vi "get setpoint.vi"(7 "error in (no error)":errorcluster, 9 "Loop":u8(ring) items=["1", "2", "3", "4"], 10 "VISA In":refnum<visa-resource-name>) -> (0 "error out":errorcluster, 1 "数字":dbl, 3 "VISA out":refnum<visa-resource-name>)   [LabVIEW 2019, in "9T cmag.lvlib"]
uses:
  9T cmag.lvlib
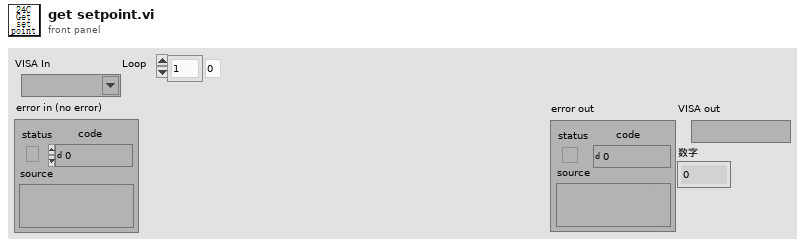
[diagram p1: front panel]
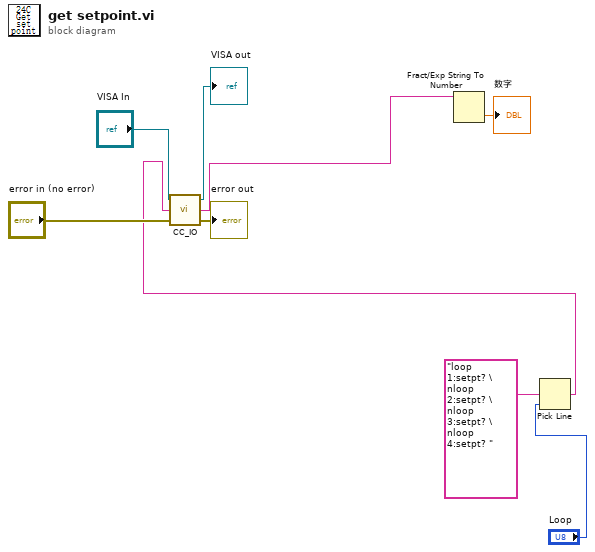
[diagram p0: block diagram]
diagram:
  n1 = Pick Line(multi-line string="loop 1:setpt? \nloop 2:setpt? \nloop 3:setpt? \nloop 4:setpt? " ("string"), line index="Loop") -> (output string=w1:string)  [unwired: 1 in]
  n2 = call "CC_IO.vi"("error in (no error)"="error in (no error)", "Output Command"=w1, "VISA In"="VISA In") -> ("error out"=→"error out":errorcluster, "Input String"=w5:string, "VISA out"=→"VISA out":refnum<visa-resource-name>)
  n3 = Fract/Exp String To Number(string=w5) -> (number=→"数字":dbl)  [unwired: 3 in, 1 out]
